vi "DLL Log Control.vi"(8 "error in":errorcluster, 10 "File Path":string, 11 "DllLogActions":T1) -> (0 "error out":errorcluster)   [LabVIEW 2013]
uses:
  DLL Log Actions.ctl
  C:/Users/mbletzin/Desktop/Work/NewLbcbConversionDll/DLL/LbcbConversions.dll
  DLL/LbcbConversions.dll
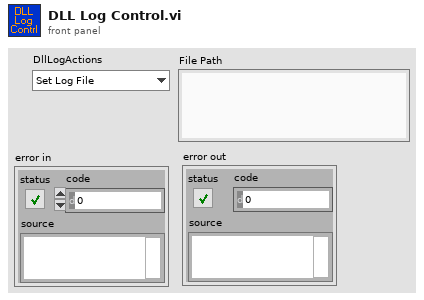
[diagram p1: front panel]
types:
  T1 = typedef "DLL Log Actions.ctl" = enum16{"Set Log File", "Set Log Config File", "Init"}
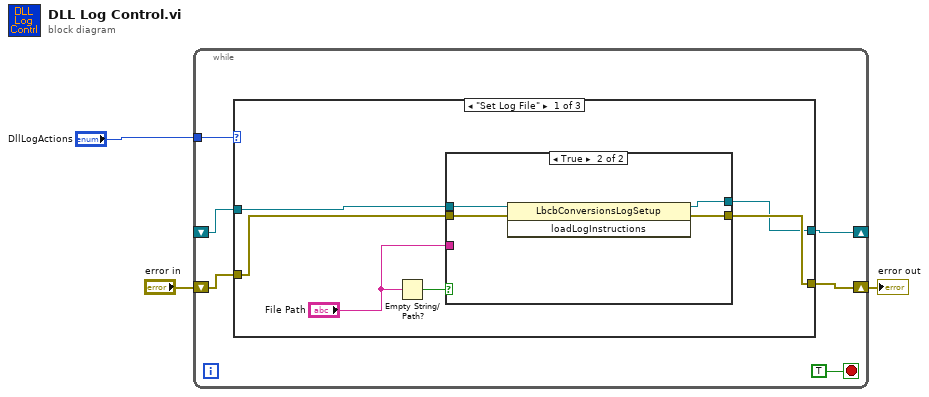
[diagram p0: block diagram]
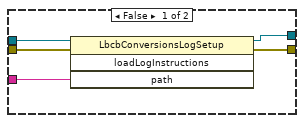
[diagram p2: hidden frame]
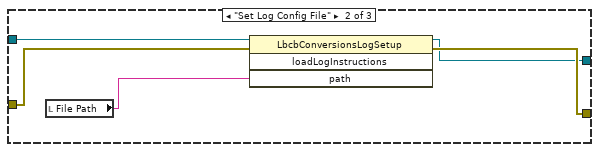
[diagram p3: hidden frame]
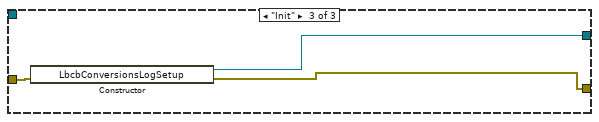
[diagram p4: hidden frame]
diagram:
  n1 = while {
    shift-right: [w9] -> _
    shift-left: _ -> [w4]
    shift-right: [w8] -> w1
    shift-left: "error in" -> [w6]
    tunnel: "DllLogActions" -> [w5]
    stop <- TRUE stop-if-true
    n2 = case shown="\"Set Log File\"" w5 {
      tunnel: [w12 w26 w31] -> w9
      tunnel: [w14 w28 w30] -> w8
      tunnel: w6 -> [w15 w29 w32]
      tunnel: w4 -> [w13 w27 _]
      frame "Set Log File" {
        n3 = Empty String/Path?(string/path="File Path") -> (empty?=w11:bool)
        n4 = case shown="True" w11 {
          tunnel: w15 -> [w20 w24]
          tunnel: [w19 w23] -> w14
          tunnel: w13 -> [w18 w22]
          tunnel: [w17 w21] -> w12
          tunnel: "File Path" -> [w16 _]
          frame False {
            n5 = invoke class="LbcbConversionsLogSetup" method="loadLogInstructions"(reference=w18, error in=w20, "path"=w16) -> (reference out=w17:refnum<k24>, error out=w19:errorcluster)  [unwired: 1 in, 2 out]
          }
          frame True {
            n6 = invoke class="LbcbConversionsLogSetup" method="loadLogInstructions"(reference=w22, error in=w24) -> (reference out=w21:refnum<k24>, error out=w23:errorcluster)  [unwired: 1 in, 1 out]
          }
        }
      }
      frame "Set Log Config File" {
        n7 = local read "File Path"() -> (w25:string)
        n8 = invoke class="LbcbConversionsLogSetup" method="loadLogInstructions"(reference=w27, error in=w29, "path"=w25) -> (reference out=w26:refnum<k24>, error out=w28:errorcluster)  [unwired: 1 in, 2 out]
      }
      frame "Init" {
        n9 = constructor class="LbcbConversionsLogSetup"(error in=w32) -> (reference out=w31:refnum<k24>, error out=w30:errorcluster)  [unwired: 2 in, 1 out]
      }
    }
  }
  "error out" <- w1
